vi "Load Config List.vi"() -> (0 "Config Names":string[](array[string]), 2 "StringsAndValues[]":T1(array[cluster]), 3 "Config File Paths":path[](array[path]))   [LabVIEW 2023]
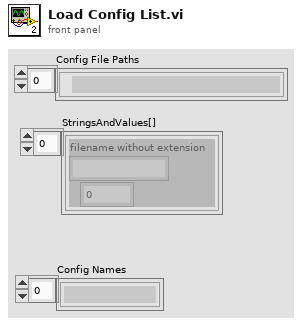
[diagram p1: front panel]
types:
  T1 = cluster{"filename without extension":string, i32}[]
  T2 = cluster{"filename without extension":string, i32}
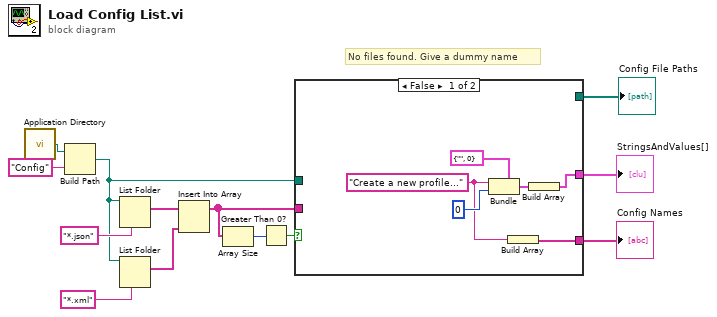
[diagram p0: block diagram]
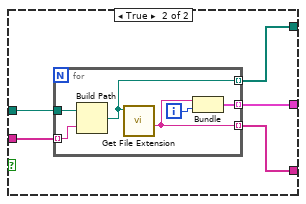
[diagram p2: hidden frame]
diagram:
  # "No files found. Give a dummy name"
  n1 = call <vilib>:"Application Directory.vi"() -> ("Application Directory"=w11:path)
  n2 = Build Path(base path=w11, name or relative path="Config") -> (appended path=w4:path)
  n3 = List Folder(path=w4, pattern="*.json") -> (filenames=w6:string[])  [unwired: 2 in, 3 out]
  n4 = List Folder(path=w4, pattern="*.xml") -> (filenames=w5:string[])  [unwired: 2 in, 3 out]
  n5 = Insert Into Array(array=w6, new element=w5) -> (w3:string[])  [unwired: 1 in]
  n6 = Array Size(array=w3) -> (size(s)=w2:i32)
  n7 = Greater Than 0?(x=w2) -> (x > 0?=w1:bool)
  n8 = case shown="False" w1 {
    tunnel: [w18 w24] -> w10
    tunnel: [_ w23] -> w9
    tunnel: [w15 w22] -> w8
    tunnel: w3 -> [_ w21]
    tunnel: w4 -> [_ w20]
    frame False {
      w14 = "Create a new profile..." ("pattern")
      n9 = Bundle(cluster=T2 {"filename without extension"="", 0} ("StringsAndValues[]"), "filename without extension"=w14, 0) -> (w17:T2)
      n10 = Build Array(w14) -> (w15:string[])
      n11 = Build Array(w17) -> (w18:T1)
    }
    frame True {
      n12 = for {
        tunnel: w21 -> [w29] mode=indexing
        tunnel: w20 -> [w30]
        tunnel: [w27] -> w24 mode=indexing
        tunnel: [w26] -> w23 mode=indexing
        tunnel: [w25] -> w22 mode=indexing
        i -> [w28]
        n13 = Build Path(base path=w30, name or relative path=w29) -> (appended path=w26:path)
        n14 = call <vilib>:"Get File Extension.vi"("file"=w26) -> ("filename without extension"=w25:string)  [unwired: 6 in, 4 out]
        n15 = Bundle("filename without extension"=w25, w28) -> (w27:T2)  [unwired: 1 in]
      }
    }
  }
  "StringsAndValues[]" <- w10
  "Config File Paths" <- w9
  "Config Names" <- w8
